vi "Cache_Get Path to Cache from Class Name.vi"(8 "error in (no error)":errorcluster, 11 "Class Name":string) -> (0 "error out":errorcluster, 1 "Success?":bool, 3 "Cache Path":path)   [LabVIEW 2020, in "ClassLoader.lvlib"]
uses:
  ClassLoader.lvlib
  Cache_PPL Global.vi
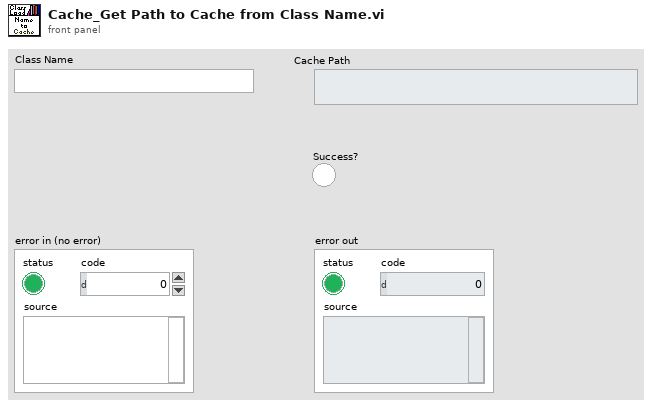
[diagram p1: front panel]
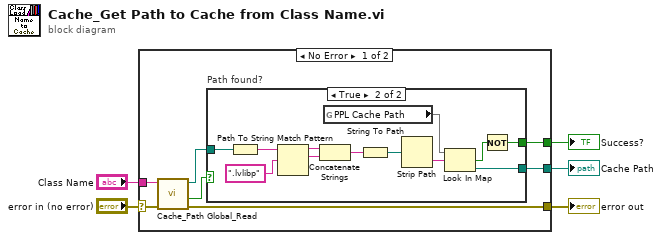
[diagram p0: block diagram]
diagram:
  n1 = case shown="No Error" "error in (no error)" {
    selector: "error in (no error)" -> [w12 w25]
    tunnel: "Class Name" -> [w11 _]
    tunnel: [w7 w25] -> w3
    tunnel: [w8 _] -> w2
    tunnel: [w6 _] -> w1
    frame No Error {
      n2 = call "Cache_Path Global_Read.vi"("error in (no error)"=w12, "Class Name"=w11) -> ("error out"=w7:errorcluster, "Success?"=w10:bool, "Class Path"=w9:path)  [unwired: 7 in]
      n3 = case "Path found?" shown="True" w10 {
        tunnel: w9 -> [_ w24]
        tunnel: [_ w14] -> w8
        tunnel: [_ w13] -> w6
        frame False {
        }
        frame True {
          n4 = Path To String(path=w24) -> (string=w23:string)
          n5 = Match Pattern(string=w23, regular expression=".lvlibp") -> (before substring=w21:string, match substring=w20:string)  [unwired: 1 in, 2 out]
          n6 = Concatenate Strings(w21, w20) -> (w19:string)
          n7 = global read "Cache_PPL Global.vi" "PPL Cache Path"() -> (w17:map{string, path})
          n8 = String To Path(string=w19) -> (path=w18:path)
          n9 = Strip Path(path=w18) -> (name=w16:string)  [unwired: 1 out]
          n10 = Look In Map(map=w17, key=w16) -> (key not found?=w15:bool, value=w13:path)  [unwired: 1 in]
          n11 = Not(x=w15) -> (.not. x?=w14:bool)
        }
      }
    }
    frame Error {
    }
  }
  "error out" <- w3
  "Success?" <- w2
  "Cache Path" <- w1
